vi "destroy queues.vi"(11 "Template in":refnum<class "Template.lvclass">) -> (3 "Template out":refnum<class "Template.lvclass">)   [LabVIEW 2020, in "Template.lvlib" / "Template.lvclass"]
doc: "Destroy the queues that were used to control the actor's behavior.\nOverride this method if you needed new queues in the application.\nCalling the parent method is <b>mandatory</b>\nThis vi is called in the Pre Launch Init override of the Actor Framework overrides."
uses:
  Template.lvclass
  Template.lvclass/Template.ctl
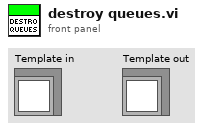
[diagram p1: front panel]
types:
  T1 = typedef "Template.lvlib/Template.lvclass/base actor queues.ctl" = cluster{"DVR Pool":refnum<queue>, "Actor's Data":refnum<queue>}
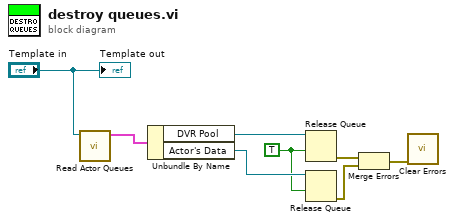
[diagram p0: block diagram]
diagram:
  w4 = TRUE ("force destroy? (F)")
  n1 = call "Read Actor Queues.vi"("Template in"="Template in") -> ("Base Actor Queues"=w7:T1)  [unwired: 10 in]
  n2 = Unbundle By Name(w7) -> ("DVR Pool"=w6:refnum<queue>, "Actor's Data"=w5:refnum<queue>)
  n3 = Release Queue(queue=w6, force destroy? (F)=w4) -> (error out=w3:errorcluster)  [unwired: 1 in, 2 out]
  n4 = Release Queue(queue=w5, force destroy? (F)=w4) -> (error out=w2:errorcluster)  [unwired: 1 in, 2 out]
  n5 = Merge Errors(w3, w2) -> (w1:errorcluster)
  n6 = call <vilib>:"Clear Errors.vi"("error in (no error)"=w1) -> ()  [unwired: 5 in, 2 out]
  "Template out" <- "Template in"
